vi "Acq-module-5761.vi"(5 "IntermediateFIFO":refnum<k21>="FIFO0", 7 "AI Cluster":T1={"FPGA AI3"="IO Module\\AI 0 Data N", "FPGA AI3 2"="IO Module\\AI 1 Data N", "FPGA AI3 3"="IO Module\\AI 2 Data N", "FPGA AI3 4"="IO Module\\AI 3 Data N"}, 8 "Nchannels":T2, 9 "SamplingRate0":u16, 11 "Cluster in":T4={0, 0, 0, 0, 0, 0, 0, TRUE, TRUE, 0, 0, 0}) -> (1 "Analog Out Cluster":T3, 3 "cluster out":T4)   [LabVIEW 2013]
uses:
  N Channels 5761.ctl
  <vilib>/rvi/DataTransferAndStorage/Container/Common/niFpgaContainerExecOnDevCompGetState.vi
  <vilib>/rvi/FIFO/Fifo_Resource/nirvififoEmulationWriteFpgaImpl.vi
  <vilib>/rvi/DataTransferAndStorage/Container/Common/niFpgaContainerGetUniqueNameForEmu.vi
  <vilib>/rvi/interface/RandomDataEmulation/nirviRandomDataFPGAFIFO.vi
  <vilib>/rvi/interface/RandomDataEmulation/niFpgaRandomDataHandleErrors.vi
  <vilib>/rvi/eio/common/nirviEmuReportErrorAndStop.vi
  <vilib>/rvi/eio/common/nirviEmuTemplateMethod_errors.vi
  <vilib>/rvi/DataTransferAndStorage/Container/XNode/niFpgaContainer.xnode
  <vilib>/rvi/FIFO/Fifo_Resource/niFpgaFifoEmulationRefIn.vi
  <vilib>/eio/EIONode/EIONode.xnode
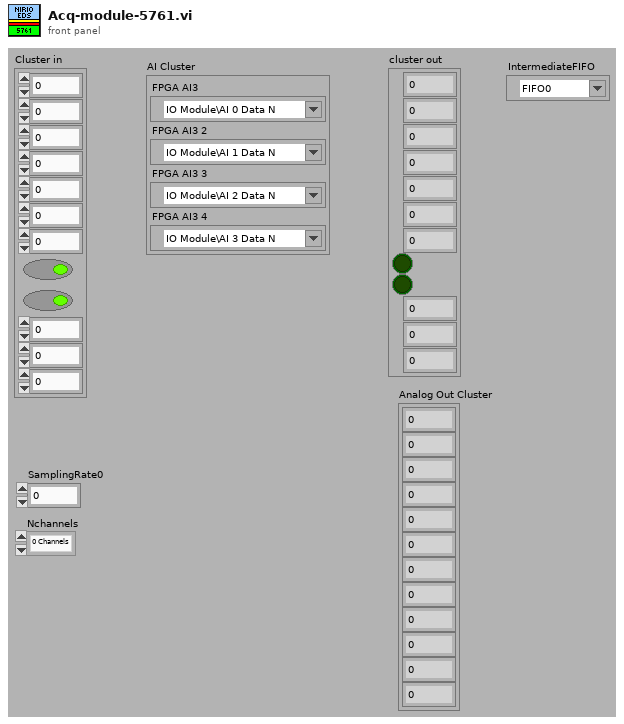
[diagram p1: front panel]
types:
  T1 = cluster{"FPGA AI3":refnum<k21>, "FPGA AI3 2":refnum<k21>, "FPGA AI3 3":refnum<k21>, "FPGA AI3 4":refnum<k21>}
  T2 = typedef "N Channels 5761.ctl" = enum16{"0 Channels", "1 Channels", "2 Channels", "3 Channels", "4 Channels", ""}
  T3 = cluster{i16, i16, i16, i16, i16, i16, i16, i16, i16, i16, i16, i16}
  T4 = cluster{u16, u16, u64, u64, u64, u64, i16, bool, bool, u64, u16, u16}
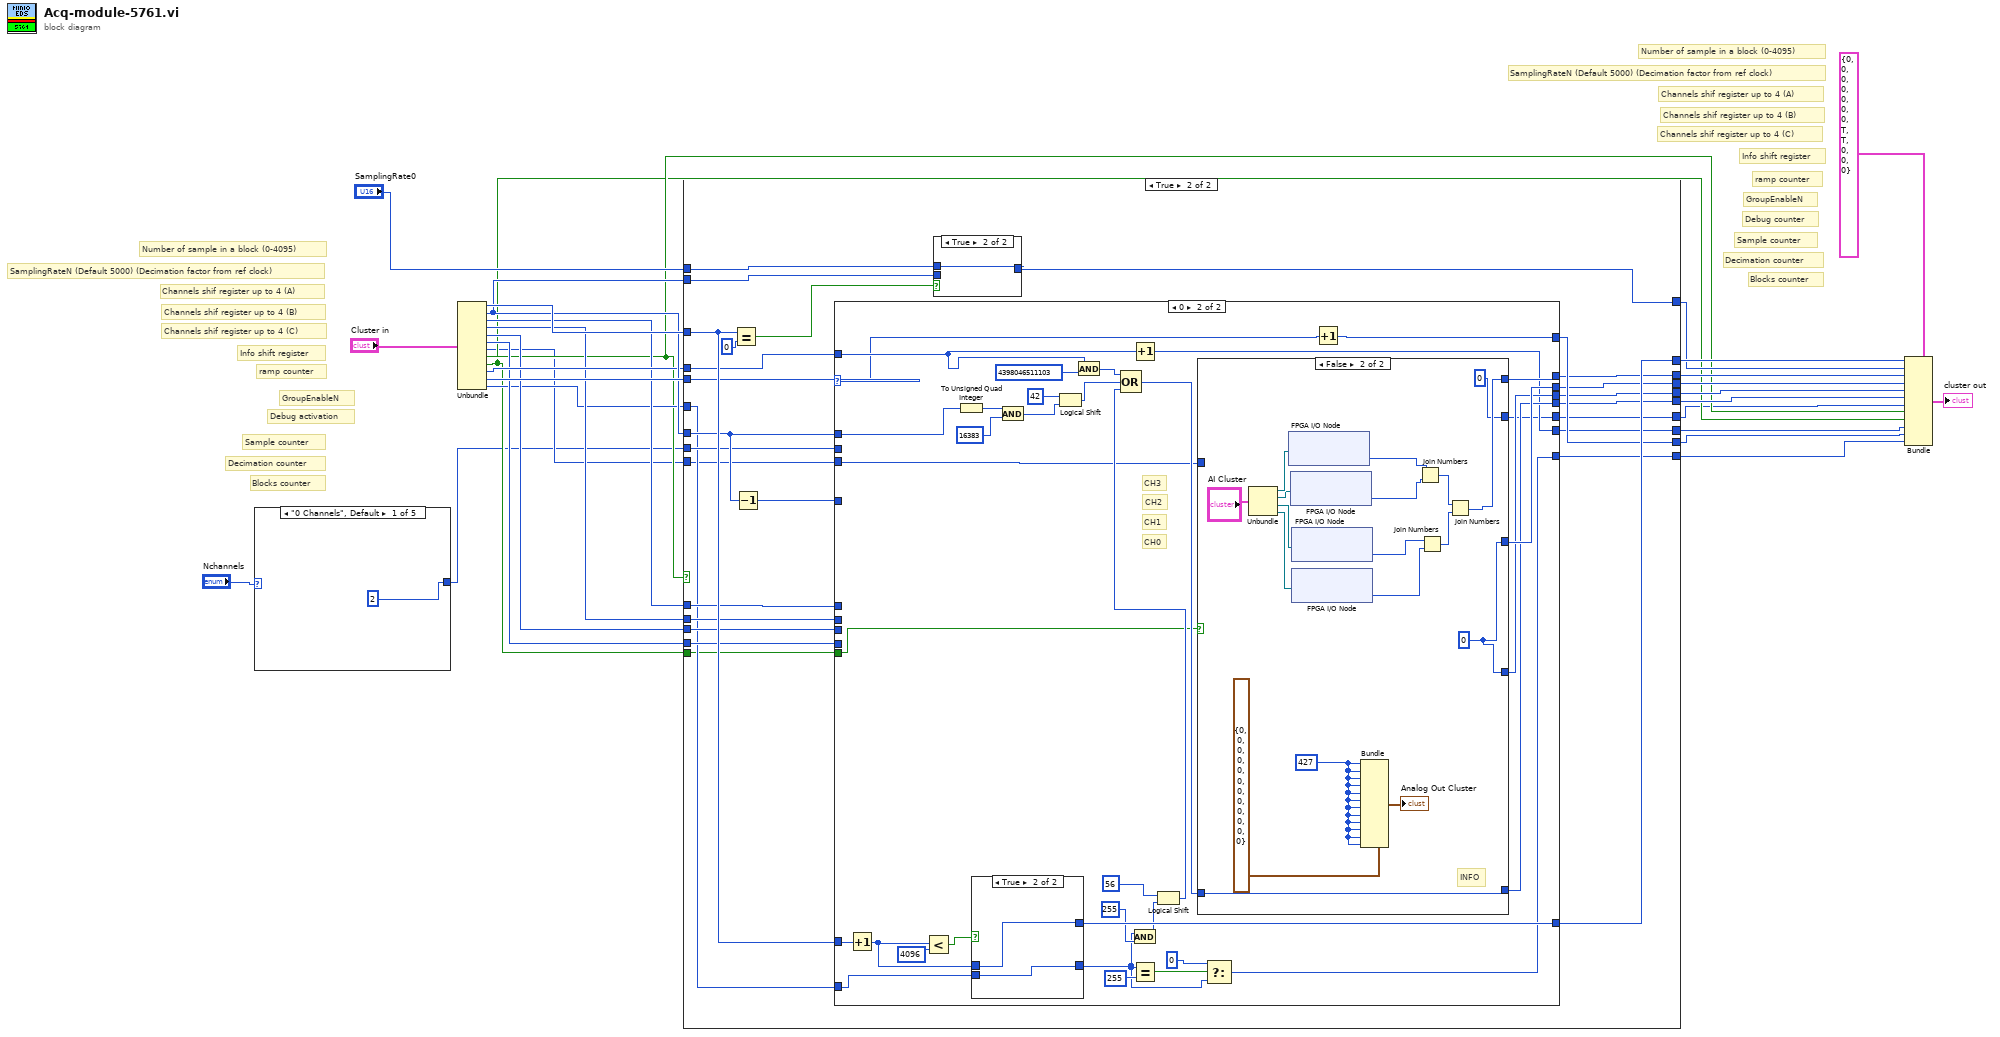
[diagram p0: block diagram]
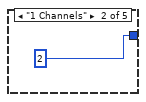
[diagram p2: hidden frame]
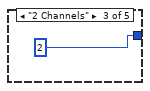
[diagram p3: hidden frame]
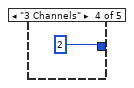
[diagram p4: hidden frame]
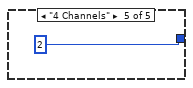
[diagram p5: hidden frame]
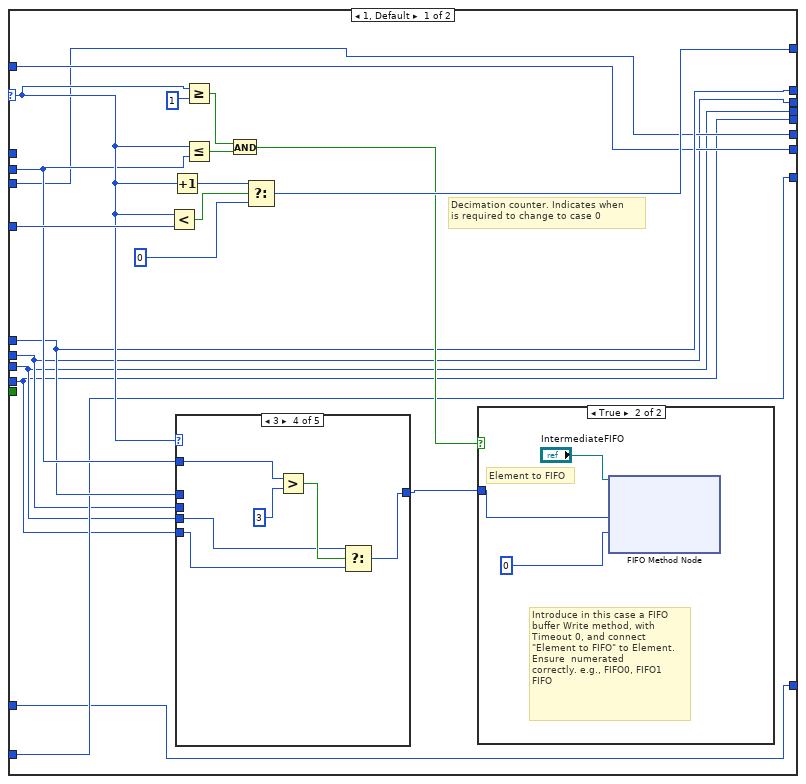
[diagram p7: hidden frame]
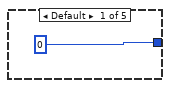
[diagram p9: hidden frame]
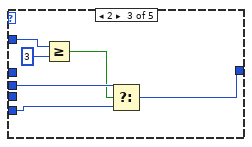
[diagram p11: hidden frame]
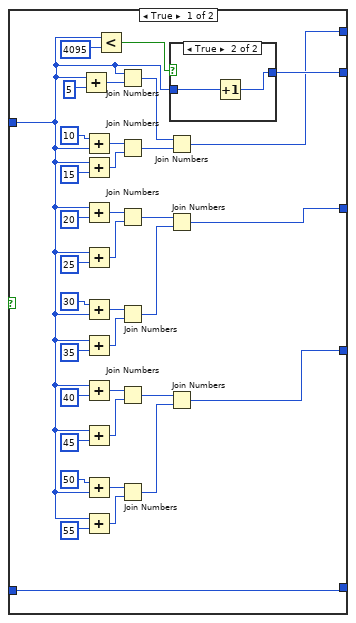
[diagram p13: hidden frame]
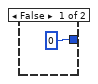
[diagram p14: hidden frame]
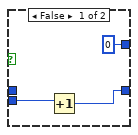
[diagram p15: hidden frame]
diagram:
  # "Blocks counter"
  # "Decimation counter"
  # "Blocks counter"
  # "Sample counter"
  # "Debug counter"
  # "ramp counter"
  # "Info shift register"
  # "Channels shif register up to 4 (C)"
  # "Channels shif register up to 4 (B)"
  # "Channels shif register up to 4 (A)"
  # "SamplingRateN (Default 5000) (Decimation factor from ref clock)"
  # "Number of sample in a block (0-4095)"
  # "GroupEnableN"
  # "Decimation counter"
  # "Sample counter"
  # "Debug activation"
  # "ramp counter"
  # "Info shift register"
  # "Channels shif register up to 4 (C)"
  # "Channels shif register up to 4 (B)"
  # "Channels shif register up to 4 (A)"
  # "SamplingRateN (Default 5000) (Decimation factor from ref clock)"
  # "Number of sample in a block (0-4095)"
  # "GroupEnableN"
  n1 = case shown="\"0 Channels\", Default" "Nchannels" {
    tunnel: [u8 2 ("Number of words") u8 2 ("Number of words") u8 2 ("Number of words") u8 2 ("Number of words") u8 2 ("Number of words")] -> w1
    frame "0 Channels", Default {
    }
    frame "1 Channels" {
    }
    frame "2 Channels" {
    }
    frame "3 Channels" {
    }
    frame "4 Channels" {
    }
  }
  n2 = Unbundle("Cluster in") -> (w28:u16, w15:u16, w12:u64, w11:u64, w10:u64, w9:u64, w4:i16, w6:bool, w5:bool, w14:u64, w21:u16, w8:u16)
  n3 = case shown="True" w6 {
    tunnel: w28 -> [w41 w66]
    tunnel: "SamplingRate0" -> [_ w69]
    tunnel: w15 -> [w42 w67]
    tunnel: [w41 w65] -> w25
    tunnel: [w42 w64] -> w24
    tunnel: w15 -> [_ w63]
    tunnel: w1 -> [_ w61]
    tunnel: w21 -> [w43 w60]
    tunnel: [w43 w59] -> w20
    tunnel: [w40 w58] -> w19
    tunnel: [w39 w57] -> w18
    tunnel: [w38 w56] -> w17
    tunnel: [w37 w55] -> w16
    tunnel: w14 -> [w36 w54]
    tunnel: [w36 w53] -> w13
    tunnel: w12 -> [w40 w52]
    tunnel: w11 -> [w39 w51]
    tunnel: w10 -> [w38 w50]
    tunnel: w9 -> [w37 w49]
    tunnel: w8 -> [w35 w48]
    tunnel: [w35 w47] -> w7
    tunnel: w5 -> [_ w46]
    tunnel: w4 -> [w34 w45]
    tunnel: [w34 w44] -> w3
    frame False {
    }
    frame True {
      n4 = Equal?(x=w66, y=u16 0) -> (x = y?=w68:bool)
      n5 = Decrement(x=w63) -> (x-1=w62:u16)
      n6 = case shown="0" w60 {
        selector: w60 -> [w82 w110]
        tunnel: w66 -> [w75 w143]
        tunnel: [w75 w139] -> w65
        tunnel: w63 -> [_ w136]
        tunnel: w62 -> [w85 _]
        tunnel: w61 -> [w81 _]
        tunnel: [w84 w109] -> w59
        tunnel: [w79 w123] -> w58
        tunnel: [w73 w122] -> w57
        tunnel: [w72 w121] -> w56
        tunnel: [w71 w120] -> w55
        tunnel: w54 -> [w77 w118]
        tunnel: [w77 w117] -> w53
        tunnel: w52 -> [w79 _]
        tunnel: w51 -> [w73 _]
        tunnel: w50 -> [w72 _]
        tunnel: w49 -> [w71 _]
        tunnel: w48 -> [w76 w116]
        tunnel: [w76 w115] -> w47
        tunnel: w46 -> [_ w114]
        tunnel: w45 -> [w74 w113]
        tunnel: [w74 w112] -> w44
        frame 1, Default {
          # "Decimation counter. Indicates when \nis required to change to case 0"
          n7 = Less?(x=w82, y=w85) -> (x < y?=w78:bool)
          n8 = Increment(x=w82) -> (x+1=w90:u16)
          n9 = case shown="3" w82 {
            tunnel: [u64 0 ("Element") w95 w98 w102 w108] -> w83
            tunnel: w79 -> [_ w95 _ _ _]
            tunnel: w73 -> [_ _ w101 _ _]
            tunnel: w72 -> [_ _ _ w104 _]
            tunnel: w71 -> [_ _ w97 w103 w108]
            tunnel: w81 -> [_ _ w100 w107 _]
            frame Default {
            }
            frame 1 {
            }
            frame 2 {
              n10 = Greater Or Equal?(x=w100, y=u8 3) -> (x >= y?=w96:bool)
              n11 = Select(t=w101, s=w96, f=w97) -> (s? t:f=w98:u64)
            }
            frame 3 {
              n12 = Greater?(x=w107, y=u8 3) -> (0:w105:bool)
              n13 = Select(t=w104, s=w105, f=w103) -> (s? t:f=w102:u64)
            }
            frame 4 {
            }
          }
          n14 = Greater Or Equal?(x=w82, y=u16 1) -> (x >= y?=w87:bool)
          n15 = Less Or Equal?(x=w82, y=w81) -> (x <= y?=w86:bool)
          n16 = And(x=w87, y=w86) -> (x .and. y?=w80:bool)
          n17 = Select(t=w90, s=w78, f=u16 0) -> (s? t:f=w84:u16)
          n18 = case shown="True" w80 {
            tunnel: w83 -> [_ w93]
            frame False {
            }
            frame True {
              # "Element to FIFO"
              # "Introduce in this case a FIFO buffer Write method, with Timeout 0, and connect \"Element to FIFO\" to Element. Ensure  numerated\ncorrectly. e.g., FIFO0, FIFO1 \nFIFO"
              n19 = xnode ("FIFO Method Node")("Element"=w93, "Timeout"=0, "FIFO In"="IntermediateFIFO") -> ()  [unwired: 2 out]
            }
          }
        }
        frame 0 {
          # "CH0"
          # "CH1"
          # "CH2"
          # "CH3"
          n20 = Increment(x=w143) -> (x+1=w140:u16)
          n21 = Less?(x=w140, y=u16 4096) -> (x < y?=w141:bool)
          n22 = To Unsigned Quad Integer(1:w136) -> (0:w138:u64)
          n23 = case shown="True" w141 {
            tunnel: w140 -> [_ w205]
            tunnel: [u16 0 w205] -> w139
            tunnel: w116 -> [w202 w204]
            tunnel: [w201 w204] -> w111
            frame False {
              n24 = Increment(x=w202) -> (x+1=w201:u16)
            }
            frame True {
            }
          }
          n25 = And(x=w138, y=i16 16383) -> (x .and. y?=w135:u64)
          n26 = Logical Shift(y=i8 42, x=w135) -> (x << y=w131:u64)
          n27 = And(x=w118, y=u64 4398046511103) -> (x .and. y?=w132:u64)
          n28 = Increment(x=w118) -> (x+1=w117:u64)
          n29 = And(x=w111, y=u64 255) -> (x .and. y?=w129:u64)
          n30 = Equal?(x=w111, y=u16 255) -> (x = y?=w126:bool)
          n31 = Logical Shift(y=i8 56, x=w129) -> (x << y=w124:u64)
          n32 = Compound Arithmetic op=OR(w132, w131, w124) -> (w119:u64)
          n33 = case shown="False" w114 {
            tunnel: [w147 w200] -> w123
            tunnel: [w146 w194] -> w122
            tunnel: [w145 w194] -> w121
            tunnel: [w144 w199] -> w120
            tunnel: w119 -> [w144 w199]
            tunnel: w113 -> [w149 _]
            tunnel: [w148 i16 0] -> w112
            frame True {
              n34 = Add(x=w149, y=i16 5) -> (x+y=w176:i16)
              n35 = Add(x=i16 10, y=w149) -> (x+y=w174:i16)
              n36 = Add(x=w149, y=i16 15) -> (x+y=w172:i16)
              n37 = Add(x=w149, y=i16 20) -> (x+y=w161:i16)
              n38 = Add(x=w149, y=i16 25) -> (x+y=w166:i16)
              n39 = Add(x=i16 30, y=w149) -> (x+y=w164:i16)
              n40 = Add(x=w149, y=i16 35) -> (x+y=w162:i16)
              n41 = Add(x=w149, y=i16 40) -> (x+y=w151:i16)
              n42 = Add(x=w149, y=i16 45) -> (x+y=w156:i16)
              n43 = Add(x=i16 50, y=w149) -> (x+y=w154:i16)
              n44 = Add(x=w149, y=i16 55) -> (x+y=w152:i16)
              n45 = Less?(x=w149, y=i16 4095) -> (x < y?=w170:bool)
              n46 = Join Numbers(hi=w149, lo=w176) -> ((hi.lo)=w179:u32)
              n47 = Join Numbers(hi=w174, lo=w172) -> ((hi.lo)=w178:u32)
              n48 = Join Numbers(hi=w161, lo=w166) -> ((hi.lo)=w169:u32)
              n49 = Join Numbers(hi=w164, lo=w162) -> ((hi.lo)=w168:u32)
              n50 = Join Numbers(hi=w151, lo=w156) -> ((hi.lo)=w159:u32)
              n51 = Join Numbers(hi=w154, lo=w152) -> ((hi.lo)=w158:u32)
              n52 = Join Numbers(hi=w179, lo=w178) -> ((hi.lo)=w147:u64)
              n53 = Join Numbers(hi=w169, lo=w168) -> ((hi.lo)=w146:u64)
              n54 = Join Numbers(hi=w159, lo=w158) -> ((hi.lo)=w145:u64)
              n55 = case shown="True" w170 {
                tunnel: w149 -> [_ w182]
                tunnel: [i16 0 w181] -> w148
                frame False {
                }
                frame True {
                  n56 = Increment(x=w182) -> (x+1=w181:i16)
                }
              }
            }
            frame False {
              w194 = 0 ("Timeout")
              w196 = i16 427
              # "INFO"
              n57 = Unbundle("AI Cluster") -> ("FPGA AI3"=w190:refnum<k21>, "FPGA AI3 2"=w188:refnum<k21>, "FPGA AI3 3"=w187:refnum<k21>, "FPGA AI3 4"=w186:refnum<k21>)
              n58 = xnode "FPGA I/O Node"("FPGA I/O In"=w190) -> ("I/O Item"=w189:i16)  [unwired: 1 out]
              n59 = xnode "FPGA I/O Node"("FPGA I/O In"=w188) -> ("I/O Item"=w185:i16)  [unwired: 1 out]
              n60 = xnode "FPGA I/O Node"("FPGA I/O In"=w187) -> ("I/O Item"=w184:i16)  [unwired: 1 out]
              n61 = xnode "FPGA I/O Node"("FPGA I/O In"=w186) -> ("I/O Item"=w183:i16)  [unwired: 1 out]
              n62 = Bundle(cluster=T3 {0, 0, 0, 0, 0, 0, 0, 0, 0, 0, 0, 0} ("Cluster 2"), w196, w196, w196, w196, w196, w196, w196, w196, w196, w196, w196, w196) -> (→"Analog Out Cluster":T3)
              n63 = Join Numbers(hi=w189, lo=w185) -> ((hi.lo)=w192:u32)
              n64 = Join Numbers(hi=w184, lo=w183) -> ((hi.lo)=w193:u32)
              n65 = Join Numbers(hi=w192, lo=w193) -> ((hi.lo)=w200:u64)
            }
          }
          n66 = Select(t=u16 0, s=w126, f=w111) -> (s? t:f=w115:u16)
          n67 = Increment(x=w110) -> (x+1=w109:u16)
        }
      }
      n68 = case shown="True" w68 {
        tunnel: w69 -> [_ w207]
        tunnel: [w206 w207] -> w64
        tunnel: w67 -> [w206 _]
        frame False {
        }
        frame True {
        }
      }
    }
  }
  n69 = Bundle(cluster=T4 {0, 0, 0, 0, 0, 0, 0, TRUE, TRUE, 0, 0, 0} ("Cluster in"), w25, w24, w19, w18, w17, w16, w3, w6, w5, w13, w20, w7) -> (→"cluster out":T4)
